vi "ReadRegister.vi"(3 "Data":u32, 4 "Offset":u32=8, 5 "error in (no error)":errorcluster) -> (0 "error out":errorcluster, 1 "Return":i32)   [LabVIEW 2015]
uses:
  BC637PCI.dll
panel:
  out "Numeric 2":dbl
  out "Numeric":dbl
  out "Data":string
  out "Offset":string
  # "Decimal"
  # "Hexidecimal"
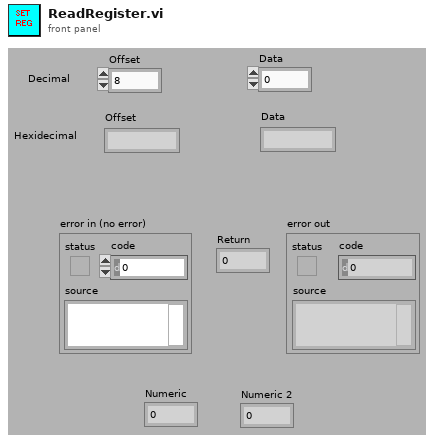
[diagram p1: front panel]
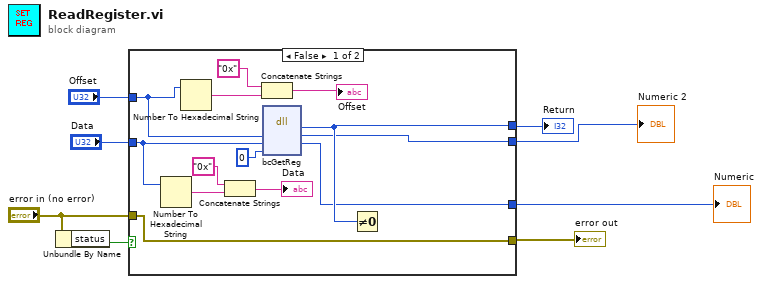
[diagram p0: block diagram]
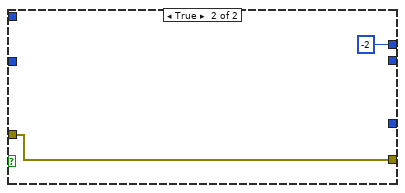
[diagram p2: hidden frame]
diagram:
  n1 = Unbundle By Name("error in (no error)") -> ("status"=w7:bool)
  n2 = case shown="False" w7 {
    tunnel: [w12 w22] -> w8
    tunnel: "error in (no error)" -> [w12 w22]
    tunnel: [w21 -2] -> w5
    tunnel: "Data" -> [w19 _]
    tunnel: "Offset" -> [w20 _]
    tunnel: [w11 _] -> w2
    tunnel: [w10 _] -> w1
    frame False {
      n3 = Number To Hexadecimal String(2:w19) -> (0:w18:string)  [unwired: 1 in]
      n4 = Number To Hexadecimal String(2:w20) -> (0:w15:string)  [unwired: 1 in]
      n5 = Concatenate Strings("0x", w18) -> (→"Data":string)
      n6 = Concatenate Strings("0x", w15) -> (→"Offset":string)
      n7 = dll-call lib="C:/GSCS 2.0/GSCS/Systems/SIcamera_Control/GPS_Drivers/BC637PCI.dll" fn="bcGetReg"("maj"=w20, "min"=w19, "nano"=0) -> ("return type"=w21:i32, "maj"=w11:u32, "min"=w10:u32)  [unwired: 4 in, 2 out]
      n8 = Not Equal To 0?(x=w21) -> ()  [unwired: 1 out]
    }
    frame True {
    }
  }
  "error out" <- w8
  "Return" <- w5
  "Numeric" <- w1
  "Numeric 2" <- w2
